vi "Write Address.vi"(8 "error in (no error)":errorcluster, 10 "Address":string, 11 "Micron Hyperion Driver in":refnum<class "Micron Hyperion Driver.lvclass">) -> (0 "error out":errorcluster, 3 "Micron Hyperion Driver out":refnum<class "Micron Hyperion Driver.lvclass">)   [LabVIEW 2016, in "Micron Hyperion Driver.lvclass"]
uses:
  Micron Hyperion Driver.lvclass
  Micron Hyperion Driver.lvclass/Micron Hyperion Driver.ctl
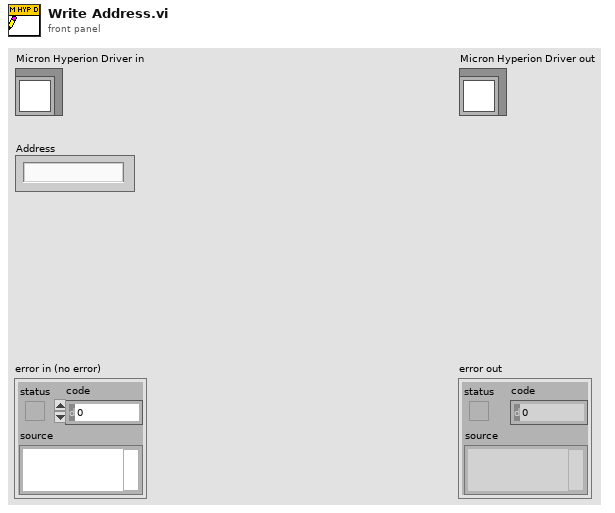
[diagram p1: front panel]
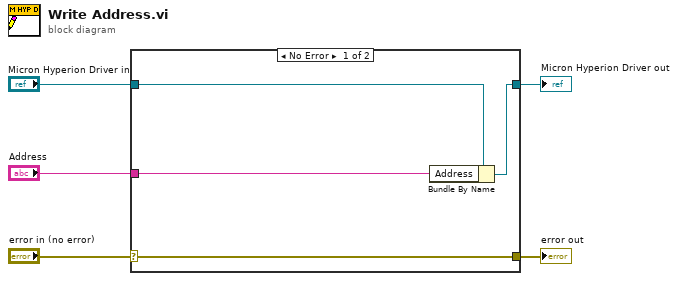
[diagram p0: block diagram]
diagram:
  n1 = case shown="No Error" "error in (no error)" {
    selector: "error in (no error)" -> [w9 w10]
    tunnel: [w9 w10] -> w4
    tunnel: [w7 w11] -> w2
    tunnel: "Micron Hyperion Driver in" -> [w8 w11]
    tunnel: "Address" -> [w6 _]
    frame No Error {
      n2 = Bundle By Name(cluster=w8, "Address"=w6) -> (w7:refnum<class "Micron Hyperion Driver.lvclass">)
    }
    frame Error {
    }
  }
  "error out" <- w4
  "Micron Hyperion Driver out" <- w2
